vi "Read Boolean Configuration.vi"(8 "error in (no error)":errorcluster, 9 "Default If Not Found":bool, 10 "Name":string, 11 "IniFileSection in":refnum<class "IniFileSection.lvclass">) -> (0 "error out":errorcluster, 1 "Not Found?":bool, 2 "Value":bool, 3 "IniFileSection out":refnum<class "IniFileSection.lvclass">)   [LabVIEW 2019, in "IniFileSection.lvclass"]
uses:
  <vilib>/gpm_packages/@cs/Configuration/Source/IniFileSection/IniFileSection.lvclass
  <vilib>/gpm_packages/@cs/Configuration/Source/IniFileSection/IniFileSection.lvclass/IniFileSection.ctl
  <vilib>/Utility/config.llb/NI_LVConfig.lvlib
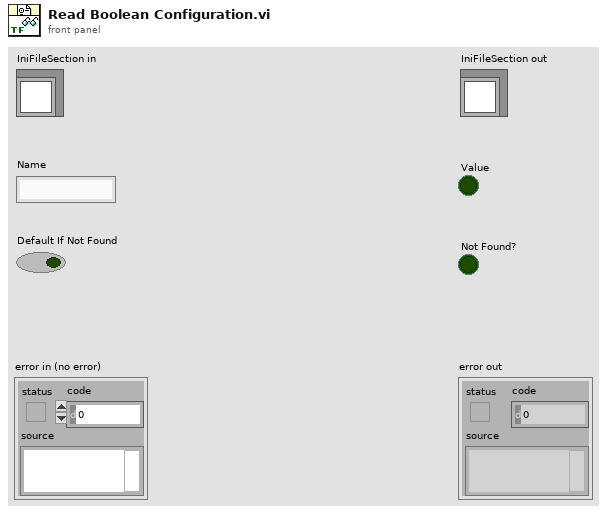
[diagram p1: front panel]
types:
  T1 = typedef "NI_LVConfig.lvlib/Config Data RefNum.ctl" = refnum<k1>
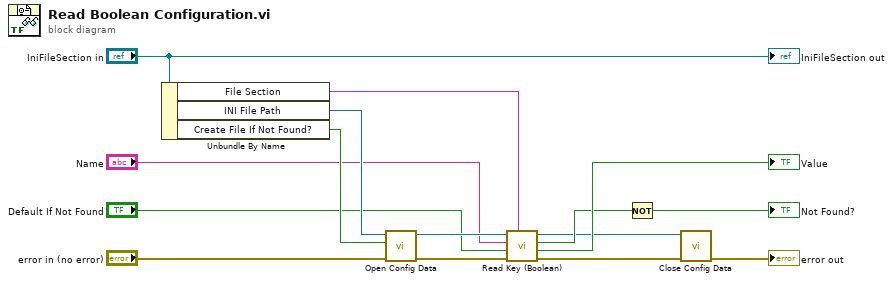
[diagram p0: block diagram]
diagram:
  n1 = Unbundle By Name("IniFileSection in") -> ("File Section"=w4:string, "INI File Path"=w15:path, "Create File If Not Found?"=w10:bool)
  n2 = call <vilib>:"Open Config Data.vi"("error in (no error)"="error in (no error)", "create file if necessary (T)"=w10, "configuration file path"=w15) -> ("error out"=w9:errorcluster, "refnum"=w3:T1)  [unwired: 6 in, 1 out]
  n3 = call <vilib>:"Read Key (Boolean).vi"("section"=w4, "error in (no error)"=w9, "default value"="Default If Not Found", "key"="Name", "refnum"=w3) -> ("error out"=w8:errorcluster, "value"=→"Value":bool, "found?"=w6:bool, "refnum out"=w5:T1)  [unwired: 3 in]
  n4 = Not(x=w6) -> (.not. x?=→"Not Found?":bool)
  n5 = call <vilib>:"Close Config Data.vi"("error in (no error)"=w8, "refnum"=w5) -> ("error out"=→"error out":errorcluster)  [unwired: 8 in, 1 out]
  "IniFileSection out" <- "IniFileSection in"
